vi "Send Channel Config.vi"(8 "error in (no error)":errorcluster, 9 "Flow Name":string, 10 "Asset Name":string, 11 "Sift Client in":refnum<class "Sift Client.lvclass">) -> (0 "error out":errorcluster, 3 "Sift Client out":refnum<class "Sift Client.lvclass">)   [LabVIEW 2024, in "Sift Client.lvlib" / "Sift Client.lvclass"]
uses:
  Sift Client.lvclass
  Generate Sift Protos/SiftProxy_client/RPC Messages/sift_proxy_v1_CreateLabviewIngestionConfigRequest_Flat.ctl
  Generate Sift Protos/SiftProxy_client/RPC Messages/sift_proxy_v1_ChannelConfig_Flat.ctl
  Generate Sift Protos/SiftProxy_client/RPC Messages/sift_proxy_v1_ChannelDataType.ctl
  Generate Sift Protos/SiftProxy_client/RPC Messages/sift_proxy_v1_ChannelEnumType_Flat.ctl
  Generate Sift Protos/SiftProxy_client/RPC Messages/sift_proxy_v1_ChannelBitFieldElement_Flat.ctl
  Sift Client.lvclass/Sift Client.ctl
  <vilib>/Utility/error.llb/Error Cluster From Error Code.vi
  <vilib>/ErrorRing/Error Ring.xnode
  Generate Sift Protos/SiftProxy_client/SiftProxy_client.lvlib
panel:
  in  "CreateLabviewIngestionConfigRequest":T1
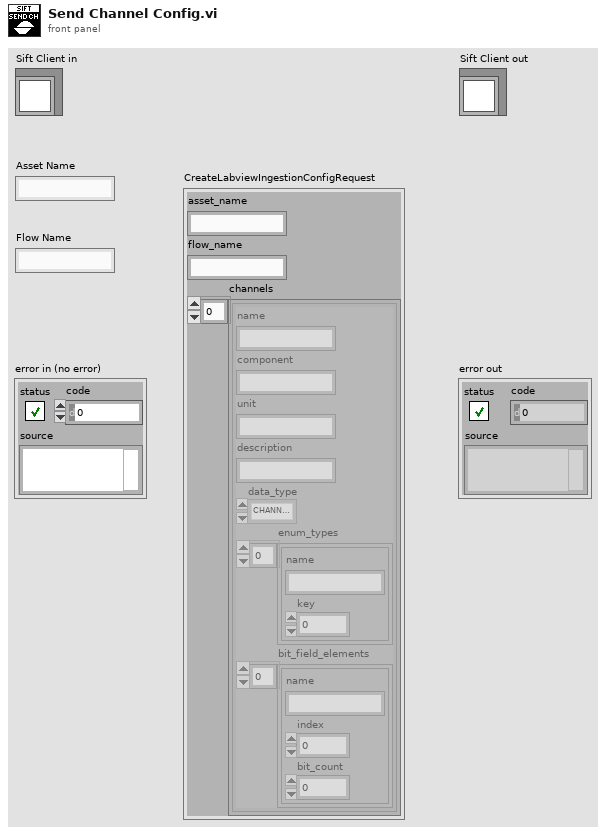
[diagram p1: front panel]
types:
  T1 = typedef "SiftProxy_client.lvlib/sift_proxy_v1_CreateLabviewIngestionConfigRequest_Flat.ctl" = cluster{"asset_name":string, "flow_name":string, "channels":T2[]}
  T2 = typedef "SiftProxy_client.lvlib/sift_proxy_v1_ChannelConfig_Flat.ctl" = cluster{"name":string, "component":string, "unit":string, "description":string, "data_type":T3, "enum_types":T4[], "bit_field_elements":T5[]}
  T3 = typedef "SiftProxy_client.lvlib/sift_proxy_v1_ChannelDataType.ctl" = enum32{"CHANNEL_DATA_TYPE_UNSPECIFIED", "CHANNEL_DATA_TYPE_DOUBLE", "CHANNEL_DATA_TYPE_STRING", "CHANNEL_DATA_TYPE_ENUM", "CHANNEL_DATA_TYPE_BIT_FIELD", "CHANNEL_DATA_TYPE_BOOL", "CHANNEL_DATA_TYPE_FLOAT", "CHANNEL_DATA_TYPE_INT_32", "CHANNEL_DATA_TYPE_UINT_32", "CHANNEL_DATA_TYPE_INT_64", "CHANNEL_DATA_TYPE_UINT_64"}
  T4 = typedef "SiftProxy_client.lvlib/sift_proxy_v1_ChannelEnumType_Flat.ctl" = cluster{"name":string, "key":u32}
  T5 = typedef "SiftProxy_client.lvlib/sift_proxy_v1_ChannelBitFieldElement_Flat.ctl" = cluster{"name":string, "index":i32, "bit_count":u32}
  T6 = typedef "SiftProxy_client.lvlib/sift_proxy_v1_ChannelConfig.ctl" = cluster{"name":string, "component":string, "unit":string, "description":string, "data_type":T3, "enum_types":T7[], "bit_field_elements":T8[]}
  T7 = typedef "SiftProxy_client.lvlib/sift_proxy_v1_ChannelEnumType.ctl" = cluster{"name":string, "key":u32}
  T8 = typedef "SiftProxy_client.lvlib/sift_proxy_v1_ChannelBitFieldElement.ctl" = cluster{"name":string, "index":i32, "bit_count":u32}
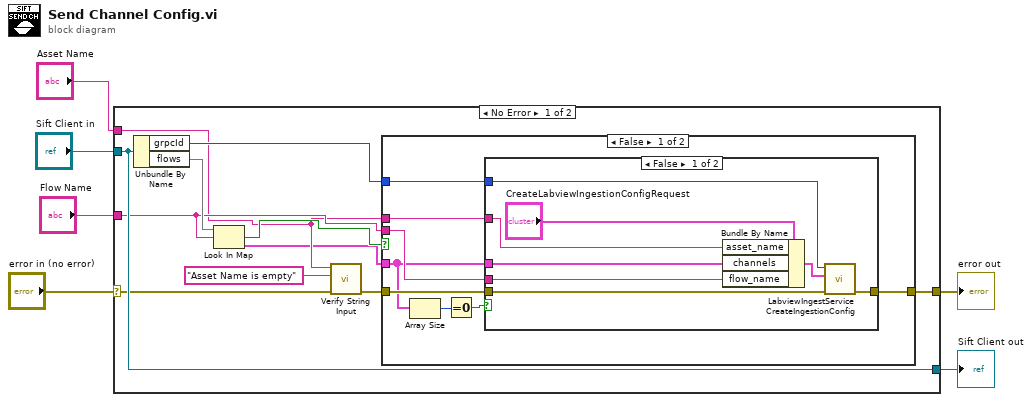
[diagram p0: block diagram]
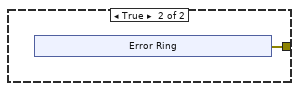
[diagram p2: hidden frame]
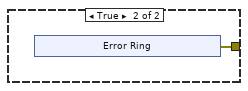
[diagram p3: hidden frame]
diagram:
  n1 = case shown="No Error" "error in (no error)" {
    selector: "error in (no error)" -> [w9 w47]
    tunnel: [w16 w47] -> w5
    tunnel: [w15 w46] -> w3
    tunnel: "Sift Client in" -> [w15 w46]
    tunnel: "Asset Name" -> [w11 _]
    tunnel: "Flow Name" -> [w13 _]
    frame No Error {
      n2 = Unbundle By Name(w15) -> ("grpcId"=w17:u64, "flows"=w14:map{string, T6[]})
      n3 = Look In Map(map=w14, key=w13) -> (key not found?=w12:bool, value=w7:T6[])  [unwired: 1 in]
      n4 = call "Verify String Input.vi"("error in (no error)"=w9, "Error Message"="Asset Name is empty", "Input"=w11) -> ("error out"=w8:errorcluster)  [unwired: 7 in, 1 out]
      n5 = case shown="False" w12 {
        tunnel: w11 -> [w25 _]
        tunnel: w17 -> [w24 _]
        tunnel: w8 -> [w23 _]
        tunnel: [w22 w40] -> w16
        tunnel: w13 -> [w21 _]
        tunnel: w7 -> [w19 _]
        frame False {
          n6 = Array Size(array=w19) -> (size(s)=w20:i32)
          n7 = Equal To 0?(x=w20) -> (x = 0?=w18:bool)
          n8 = case shown="False" w18 {
            tunnel: w25 -> [w32 _]
            tunnel: w24 -> [w30 _]
            tunnel: w23 -> [w29 _]
            tunnel: [w28 w34] -> w22
            tunnel: w21 -> [w27 _]
            tunnel: w19 -> [w26 _]
            frame False {
              n9 = Bundle By Name(cluster="CreateLabviewIngestionConfigRequest", "asset_name"=w32, "channels"=w26, "flow_name"=w27) -> (w31:T1)
              n10 = call "LabviewIngestService CreateIngestionConfig.vi"("error in"=w29, "Request Data"=w31, "gRPC ID"=w30) -> ("error out"=w28:errorcluster)  [unwired: 6 in, 2 out]
            }
            frame True {
              n11 = xnode "Error Ring"() -> ("error out"=w34:errorcluster)
            }
          }
        }
        frame True {
          n12 = xnode "Error Ring"() -> ("error out"=w40:errorcluster)
        }
      }
    }
    frame Error {
    }
  }
  "error out" <- w5
  "Sift Client out" <- w3
